vi "start daemon.vi"(8 "error in (no error)":errorcluster) -> (0 "error out":errorcluster)   [LabVIEW 2016, in "数据传输系统-06.lvlib" / "update.lvlib"]
uses:
  update.lvlib
panel:
  out "standard error":string caption="标准错误"
  out "standard output":string caption="标准输出"
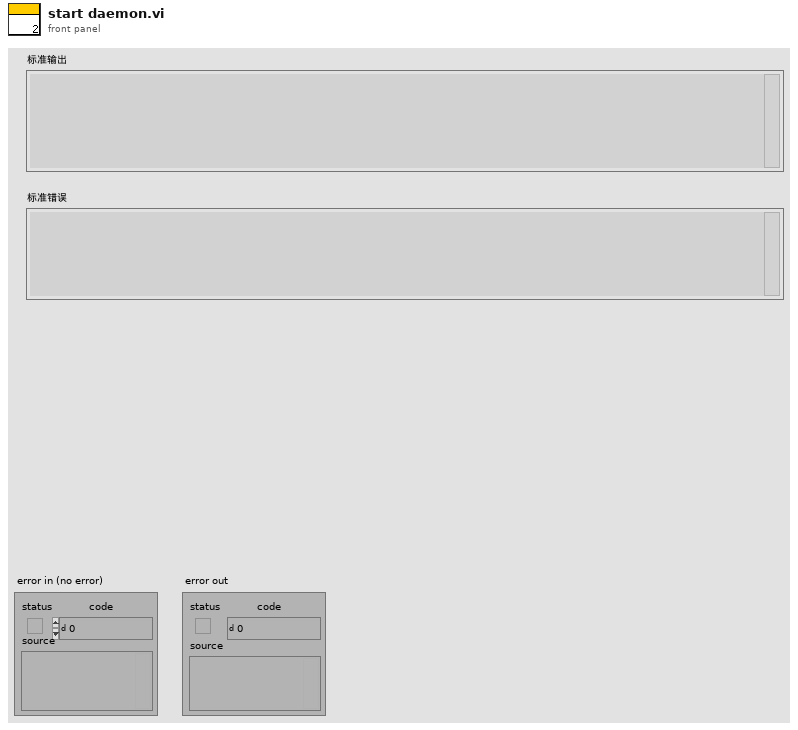
[diagram p1: front panel]
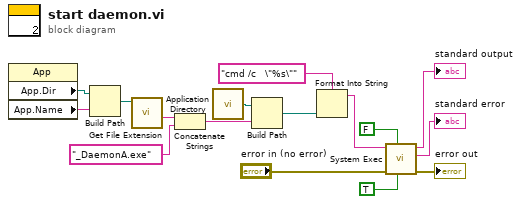
[diagram p0: block diagram]
diagram:
  n1 = property class="App"() -> ("App.Dir"=w3:path, "App.Name"=w2:string)  [unwired: 2 in, 2 out]
  n2 = Build Path(base path=w3, name or relative path=w2) -> (appended path=w1:path)
  n3 = call <vilib>:"Get File Extension.vi"("file"=w1) -> ("filename without extension"=w14:string)  [unwired: 6 in, 4 out]
  n4 = Concatenate Strings(w14, "_DaemonA.exe" ("名称或相对路径")) -> (w6:string)
  n5 = call <vilib>:"Application Directory.vi"() -> ("Application Directory"=w7:path)
  n6 = Build Path(base path=w7, name or relative path=w6) -> (appended path=w4:path)
  n7 = Format Into String(format string="cmd /c   \"%s\"" ("格式字符串"), w4) -> (resulting string=w13:string)  [unwired: 2 in, 1 out]
  n8 = call <vilib>:"System Exec.vi"("run minimized? (F)"=TRUE, "wait until completion? (T)"=FALSE, "error in (no error)"="error in (no error)", "command line"=w13) -> ("error out"=→"error out":errorcluster, "standard error"=→"standard error":string, "standard output"=→"standard output":string)  [unwired: 4 in, 1 out]
